vi "Send Core OOB TX.vi"(8 "error in (no error)":errorcluster, 11 "CIFCorePlugin in":refnum<class "CIFCorePlugin.lvclass">) -> (0 "error out":errorcluster, 3 "CIFCorePlugin out":refnum<class "CIFCorePlugin.lvclass">)   [LabVIEW 2021, in "CIFCorePlugin.lvclass"]
uses:
  CIFCorePlugin.lvclass
  Channels/CIFChannelMng/CIFChannelMng.lvclass
  074d8088-3ad4-4fdc-9542-b009f1b06b72.vi
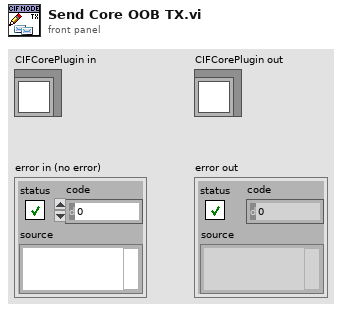
[diagram p1: front panel]
types:
  T1 = typedef "CIFCorePlugin.lvclass/Main to gRPC Data.ctl" = cluster{"Status":T2, "Plugin Overrides":T11}
  T2 = typedef "CIFCoreCommon.lvlib/Plugin Status.ctl" = cluster{"State":T3, "Timing Statistics (us)":T4, "FIFO Statistics (us)":T6, "error":T7, "Monitor Doubles":T8, "Monitor U64":T9, "Monitor I64":T10}
  T3 = typedef "CIFCoreCommon.lvlib/Plugin State.ctl" = enum32{"Null", "Creating", "Listening", "Running", "CleaningUp", "Destroying"}
  T4 = typedef "CIFCoreCommon.lvlib/Timing Statistics.ctl" = cluster{"Period":T5, "Wake Error":T5, "Execute":T5, "Housekeep":T5, "Idle":T5, "Cleanup":T5, "Custom 1 (custom units)":T5, "Custom 2 (custom units)":T5}
  T5 = typedef "CIFCoreCommon.lvlib/Timing Stats Base.ctl" = cluster{"Max":i64, "Avg":dbl, "Min":i64}
  T6 = typedef "CIFCoreCommon.lvlib/FIFO Statistics.ctl" = cluster{"From T0":T5, "From Previous Plugin":T5, "Output Error":T5}
  T7 = typedef "CIFCoreCommon.lvlib/Simple Error.ctl" = cluster{"status":bool, "code":i32}
  T8 = typedef "CIFCoreCommon.lvlib/Monitor Doubles.ctl" = cluster{"1":dbl, "2":dbl, "3":dbl, "4":dbl}
  T9 = typedef "CIFCoreCommon.lvlib/Monitor U64.ctl" = cluster{"1":u64, "2":u64, "3":u64, "4":u64}
  T10 = typedef "CIFCoreCommon.lvlib/Monitor I64.ctl" = cluster{"1":i64, "2":i64, "3":i64, "4":i64}
  T11 = typedef "CIFCoreCommon.lvlib/Plugin Overrides.ctl" = cluster{"Timing Overrides":T12}
  T12 = typedef "CIFCoreCommon.lvlib/Timing Overrides.ctl" = cluster{"Override Timing":bool, "Skip Sleep":bool, "Period (s)":dbl}
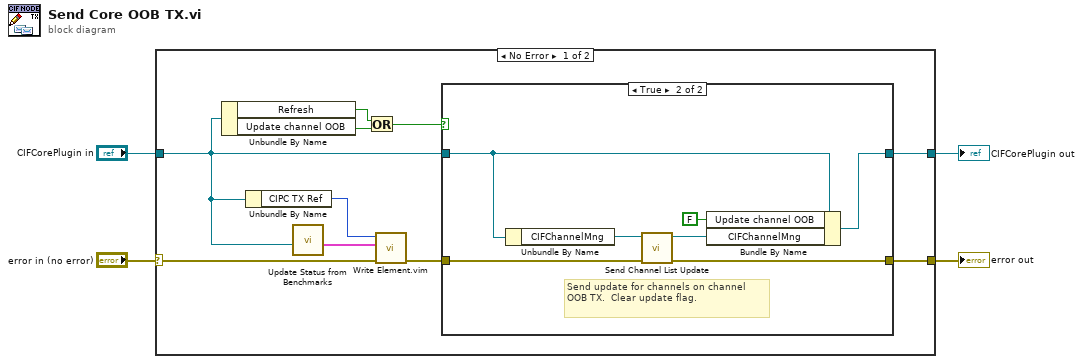
[diagram p0: block diagram]
diagram:
  n1 = case shown="No Error" "error in (no error)" {
    selector: "error in (no error)" -> [w14 w25]
    tunnel: [w13 w25] -> w2
    tunnel: [w12 w24] -> w1
    tunnel: "CIFCorePlugin in" -> [w9 w24]
    frame No Error {
      n2 = Unbundle By Name(w9) -> ("Refresh"=w8:bool, "Update channel OOB"=w7:bool)
      n3 = Unbundle By Name(w9) -> ("CIPC TX Ref"=w5:u64)
      n4 = call "Update Status from Benchmarks.vi"("CIFCorePlugin in"=w9) -> ("Main to gRPC Data"=w11:T1)  [unwired: 10 in]
      n5 = Or(x=w8, y=w7) -> (x .or. y?=w6:bool)
      n6 = call "Write Element.vim"("error in (no error)"=w14, "Data in"=w11, "CIPC Reference in"=w5) -> ("error out"=w10:errorcluster)  [unwired: 5 in, 3 out]
      n7 = case shown="True" w6 {
        tunnel: [w15 w22] -> w13
        tunnel: w9 -> [w16 w19]
        tunnel: [w16 w17] -> w12
        tunnel: w10 -> [w15 w23]
        frame False {
        }
        frame True {
          # "Send update for channels on channel OOB TX.  Clear update flag."
          n8 = Unbundle By Name(w19) -> ("CIFChannelMng"=w20:refnum<class "CIFChannelMng.lvclass">)
          n9 = call "Send Channel List Update.vi"("error in (no error)"=w23, "CIFChannelMng in"=w20) -> ("error out"=w22:errorcluster, "CIFChannelMng out"=w18:refnum<class "CIFChannelMng.lvclass">)  [unwired: 8 in]
          n10 = Bundle By Name(cluster=w19, "Update channel OOB"=FALSE ("Running Internal Data.Update channel OOB"), "CIFChannelMng"=w18) -> (w17:refnum<class "CIFCorePlugin.lvclass">)
        }
      }
    }
    frame Error {
    }
  }
  "error out" <- w2
  "CIFCorePlugin out" <- w1
